vi "startUp.vi"(8 "error in (no error)":errorcluster, 10 "ScriptEvent":refnum<class "ScriptEvent.lvclass">, 11 "SingleToneAction in":refnum<class "SingleToneAction.lvclass">) -> (0 "error out":errorcluster, 3 "SingleToneAction out":refnum<class "SingleToneAction.lvclass">)   [LabVIEW 2011, in "Views.lvlib" / "ScriptEditor.lvlib" / "SingleToneAction.lvclass"]
uses:
  SingleToneAction.lvclass
  Tools/Scripting/ScriptingEvent/ScriptEvent.lvclass
  Tools/Scripting/ScriptingEvent/ScriptEvents/SingleTone/SingleTone.lvclass
  SingleToneAction.lvclass/SingleToneAction.ctl
  ActionPanel.lvclass
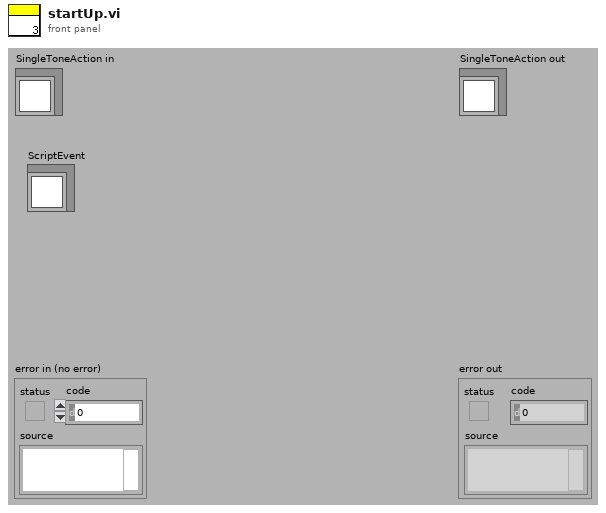
[diagram p1: front panel]
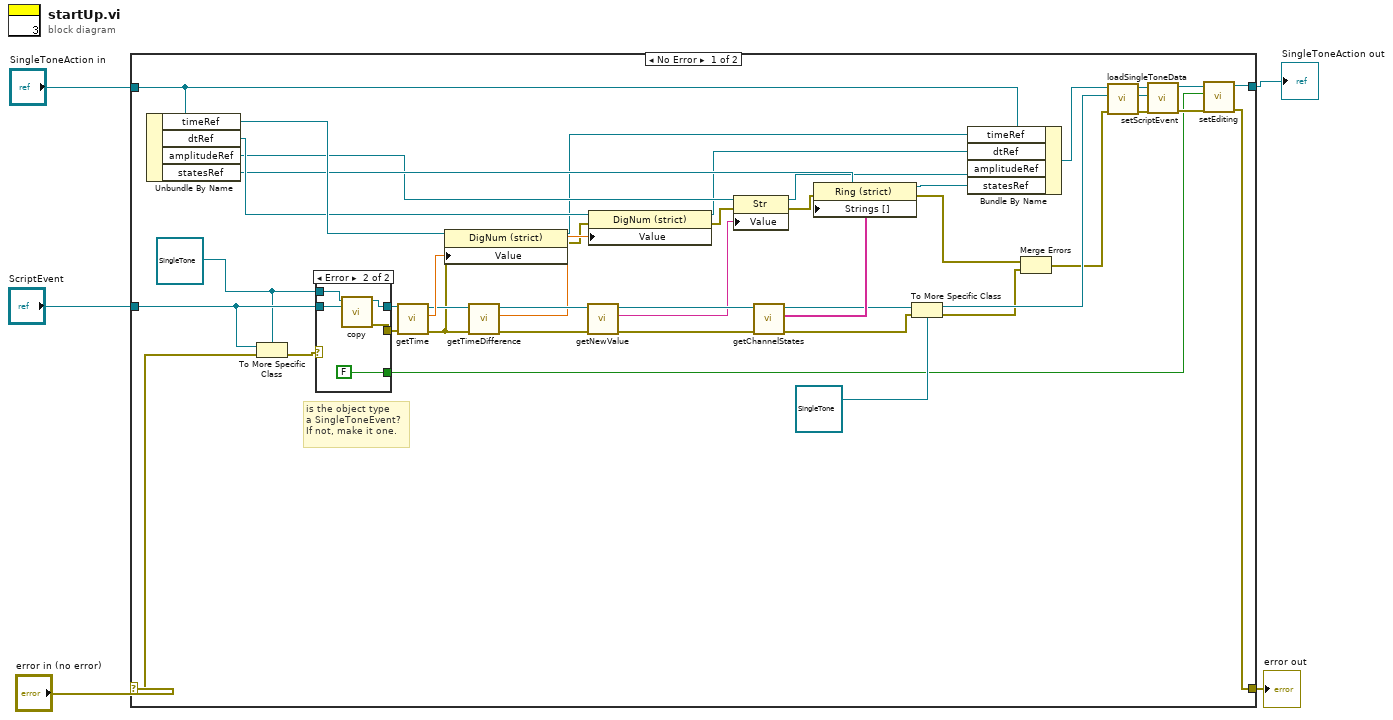
[diagram p0: block diagram]
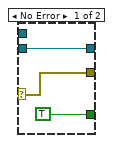
[diagram p2: hidden frame]
diagram:
  n1 = case shown="No Error" "error in (no error)" {
    selector: "error in (no error)" -> [w12 w59]
    tunnel: [w8 w59] -> w4
    tunnel: [w10 w58] -> w3
    tunnel: "SingleToneAction in" -> [w26 w58]
    tunnel: "ScriptEvent" -> [w46 _]
    frame No Error {
      w6 = refnum<class "SingleTone.lvclass"> refnum ("Tools.lvlib:Scripting.lvlib:SingleTone.lvclass")
      # "is the object type\na SingleToneEvent?\nIf not, make it one."
      n2 = Unbundle By Name(w26) -> ("timeRef"=w45:refnum<vi>, "dtRef"=w44:refnum<vi>, "amplitudeRef"=w42:refnum<vi>, "statesRef"=w43:refnum<vi>)
      n3 = To More Specific Class(target class=w6, reference=w46, error in=w12) -> (error out=w49:errorcluster)  [unwired: 1 out]
      n4 = case shown="Error" w49 {
        selector: w49 -> [w51 _]
        tunnel: w46 -> [w52 w56]
        tunnel: w6 -> [_ w57]
        tunnel: [w51 w55] -> w48
        tunnel: [w52 w54] -> w47
        tunnel: [TRUE FALSE] -> w7
        frame No Error {
        }
        frame Error {
          n5 = call-dynamic "copy.vi"("ScriptEventForCopy"=w56, "SingleTone in"=w57) -> ("error out"=w55:errorcluster, "SingleTone Copy"=w54:refnum<class "SingleTone.lvclass">)  [unwired: 8 in]
        }
      }
      n6 = call "getTime.vi"("error in (no error)"=w48, "ScriptEvent.lvclass in"=w47) -> ("error out"=w32:errorcluster, "time"=w41:dbl, "ScriptEvent.lvclass out"=w40:refnum<class "ScriptEvent.lvclass">)  [unwired: 7 in]
      n7 = property class="DigNum (strict)"(reference=w45, error in=w32, "Value"=w41) -> (reference out=w25:refnum<vi>, error out=w31:errorcluster)
      n8 = call "getTimeDifference.vi"("error in (no error)"=w32, "ScriptEvent.lvclass in"=w40) -> ("error out"=w33:errorcluster, "time difference"=w37:dbl, "ScriptEvent.lvclass out"=w39:refnum<class "ScriptEvent.lvclass">)  [unwired: 7 in]
      n9 = call "getNewValue.vi"("error in (no error)"=w33, "ScriptEvent.lvclass in"=w39) -> ("error out"=w34:errorcluster, "newValue"=w36:string, "ScriptEvent.lvclass out"=w38:refnum<class "ScriptEvent.lvclass">)  [unwired: 7 in]
      n10 = property class="DigNum (strict)"(reference=w44, error in=w31, "Value"=w37) -> (reference out=w24:refnum<vi>, error out=w30:errorcluster)
      n11 = property class="Str"(reference=w42, error in=w30, "Value"=w36) -> (reference out=w23:refnum<vi>, error out=w29:errorcluster)
      n12 = call-dynamic "getChannelStates.vi"("error in (no error)"=w34, "ScriptEvent in"=w38) -> ("error out"=w27:errorcluster, "statesValues"=w35:string[], "ScriptEvent out"=w28:refnum<class "ScriptEvent.lvclass">)  [unwired: 7 in]
      n13 = property class="Ring (strict)"(reference=w43, error in=w29, "Strings []"=w35) -> (reference out=w22:refnum<vi>, error out=w18:errorcluster)
      n14 = To More Specific Class(target class=refnum<class "SingleTone.lvclass"> refnum ("Tools.lvlib:Scripting.lvlib:SingleTone.lvclass"), reference=w28, error in=w27) -> (specific class reference=w20:refnum<class "SingleTone.lvclass">, error out=w17:errorcluster)
      n15 = Bundle By Name(cluster=w26, "timeRef"=w25, "dtRef"=w24, "amplitudeRef"=w23, "statesRef"=w22) -> (w21:refnum<class "SingleToneAction.lvclass">)
      n16 = Merge Errors(w18, w17) -> (w16:errorcluster)
      n17 = call "loadSingleToneData.vi"("error in (no error)"=w16, "SingleTone"=w20, "SingleToneAction in"=w21) -> ("error out"=w14:errorcluster, "SingleTone out"=w13:refnum<class "SingleTone.lvclass">, "SingleToneAction out"=w15:refnum<class "SingleToneAction.lvclass">)  [unwired: 6 in]
      n18 = call "setScriptEvent.vi"("error in (no error)"=w14, "ScriptEvent.lvclass"=w13, "ActionPanel.lvclass in"=w15) -> ("error out"=w9:errorcluster, "ActionPanel.lvclass out"=w11:refnum<class "SingleToneAction.lvclass">)  [unwired: 7 in]
      n19 = call "setEditing.vi"("error in (no error)"=w9, "editing?"=w7, "ActionPanel.lvclass in"=w11) -> ("error out"=w8:errorcluster, "ActionPanel.lvclass out"=w10:refnum<class "SingleToneAction.lvclass">)  [unwired: 7 in]
    }
    frame Error {
    }
  }
  "error out" <- w4
  "SingleToneAction out" <- w3
